vi "pick 1 ball new.vi"   [LabVIEW 2016, in "Test2.lvrbt"]
uses:
  Test2.lvrbt
  <vilib>/NXT/Hardware/Plugins/Tetrix DC Motor/TetrixDCMotorAddress.ctl
  <vilib>/NXT/Hardware/Plugins/Tetrix 180 deg Servo/Tetrix180ServoAddress.ctl
  <vilib>/NXT/Block Support/NXT_InputPort.ctl
  <vilib>/NXT/NXTIO Xnodes/NXTIONodeSubVIs/TETRIX IO Move Servos.vi
  <vilib>/NXT/Dual Mode Library/Waits/Wait_Num.vi
  <vilib>/NXT/NXTIO Xnodes/NXTIONodeSubVIs/TETRIX IO Move DC Motors.vi
  <vilib>/NXT/Dual Mode Library/Waits/Wait_EV3_Ultrasonic_Centimeters_Further.vi
  <vilib>/NXT/NXTIO Xnodes/NXTIONodeSubVIs/TETRIX IO Stop DC Motors.vi
  <vilib>/NXT/Dual Mode Library/Waits/Wait_EV3_Ultrasonic_Centimeter_Closer.vi
  <vilib>/NXT/NXTIO Xnodes/AddressXNode/NXTIOAddress.xnode
  <vilib>/NXT/Subs/LVHSConnector.ctl
  <vilib>/NXT/NXTIO Xnodes/NXTIOXNode/NXTIO.xnode
  <vilib>/NXT/LegoClasses/BrickReference/BrickReference.lvclass
types:
  T1 = typedef "Tetrix180ServoAddress.ctl" = i32
  T2 = cluster{"Tetrix180Servo":T1, "Tetrix180Servo":T1, "Tetrix180Servo":T1, "Tetrix180Servo":T1, "Tetrix180Servo":T1, "Tetrix180Servo":T1}
  T3 = typedef "LVHSConnector.ctl" = refnum<class "BrickReference.lvclass">
  T4 = typedef "TetrixDCMotorAddress.ctl" = i32
  T5 = typedef "NXT_InputPort.ctl" = u32
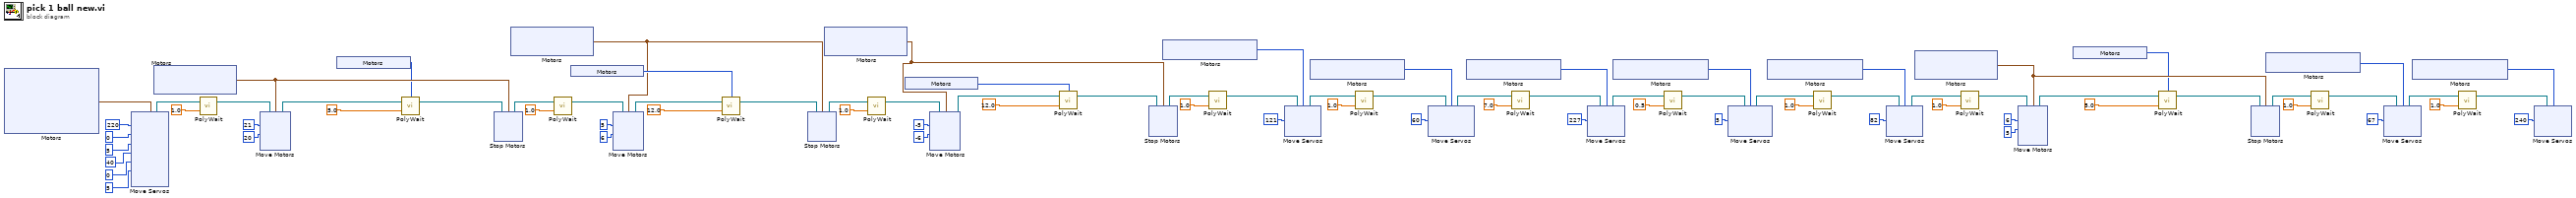
[diagram p0: block diagram]
diagram:
  n1 = xnode "Motors"() -> ("Motor"=w63:T2)
  n2 = xnode "Move Servos"("Position 6"=u8 5, "Position 5"=u8 0, "Position 4"=u8 40, "Position 3"=u8 5, "Position 2"=u8 0, "Position 1"=u8 220, "Motors"=w63) -> ("NXT/EV3"=w31:T3)  [unwired: 1 in]
  n3 = xnode "Motors"() -> ("Motor"=w33:cluster{"TetrixDCMotor":T4, "TetrixDCMotor":T4})
  n4 = call-poly <vilib>:"PolyWait.vi"("Time (1 sec)"=sgl 1.0, "NXT/EV3"=w31) -> ("NXT/EV3"=w30:T3)  [unwired: 2 in]
  n5 = xnode "Move Motors"("Power/Speed 2"=i8 20, "Power/Speed 1"=i8 21, "Motors"=w33, "NXT/EV3"=w30) -> ("NXT/EV3"=w36:T3)
  n6 = xnode "Motors"() -> ("Sensor"=w2:T5)
  n7 = call-poly <vilib>:"PolyWait.vi"("Centimeters (50)"=sgl 5.0, "NXT/EV3"=w36, "Port (Port 1)"=w2) -> ("NXT/EV3"=w34:T3)  [unwired: 1 in]
  n8 = xnode "Stop Motors"("Motors"=w33, "NXT/EV3"=w34) -> ("NXT/EV3"=w4:T3)
  n9 = xnode "Motors"() -> ("Motor"=w18:cluster{"TetrixDCMotor":T4, "TetrixDCMotor":T4})
  n10 = call-poly <vilib>:"PolyWait.vi"("Time (1 sec)"=sgl 1.0, "NXT/EV3"=w4) -> ("NXT/EV3"=w17:T3)  [unwired: 2 in]
  n11 = xnode "Motors"() -> ("Sensor"=w20:T5)
  n12 = xnode "Move Motors"("Power/Speed 2"=i8 6, "Power/Speed 1"=i8 5, "Motors"=w18, "NXT/EV3"=w17) -> ("NXT/EV3"=w22:T3)
  n13 = call-poly <vilib>:"PolyWait.vi"("Centimeters (40)"=sgl 12.0, "NXT/EV3"=w22, "Port (Port 1)"=w20) -> ("NXT/EV3"=w19:T3)  [unwired: 1 in]
  n14 = xnode "Stop Motors"("Motors"=w18, "NXT/EV3"=w19) -> ("NXT/EV3"=w16:T3)
  n15 = xnode "Motors"() -> ("Motor"=w9:cluster{"TetrixDCMotor":T4, "TetrixDCMotor":T4})
  n16 = call-poly <vilib>:"PolyWait.vi"("Time (1 sec)"=sgl 1.0, "NXT/EV3"=w16) -> ("NXT/EV3"=w12:T3)  [unwired: 2 in]
  n17 = xnode "Motors"() -> ("Sensor"=w7:T5)
  n18 = xnode "Move Motors"("Power/Speed 2"=i8 -6, "Power/Speed 1"=i8 -5, "Motors"=w9, "NXT/EV3"=w12) -> ("NXT/EV3"=w11:T3)
  n19 = call-poly <vilib>:"PolyWait.vi"("Centimeters (50)"=sgl 12.0, "NXT/EV3"=w11, "Port (Port 1)"=w7) -> ("NXT/EV3"=w10:T3)  [unwired: 1 in]
  n20 = xnode "Stop Motors"("Motors"=w9, "NXT/EV3"=w10) -> ("NXT/EV3"=w5:T3)
  n21 = xnode "Motors"() -> ("Motor"=w29:T1)
  n22 = call-poly <vilib>:"PolyWait.vi"("Time (1 sec)"=sgl 1.0, "NXT/EV3"=w5) -> ("NXT/EV3"=w3:T3)  [unwired: 2 in]
  n23 = xnode "Move Servos"("Position 1"=u8 121, "Motors"=w29, "NXT/EV3"=w3) -> ("NXT/EV3"=w27:T3)
  n24 = xnode "Motors"() -> ("Motor"=w75:T1)
  n25 = call-poly <vilib>:"PolyWait.vi"("Time (1 sec)"=sgl 1.0, "NXT/EV3"=w27) -> ("NXT/EV3"=w50:T3)  [unwired: 2 in]
  n26 = xnode "Move Servos"("Position 1"=u8 60, "Motors"=w75, "NXT/EV3"=w50) -> ("NXT/EV3"=w72:T3)
  n27 = xnode "Motors"() -> ("Motor"=w71:T1)
  n28 = call-poly <vilib>:"PolyWait.vi"("Time (1 sec)"=sgl 7.0, "NXT/EV3"=w72) -> ("NXT/EV3"=w69:T3)  [unwired: 2 in]
  n29 = xnode "Move Servos"("Position 1"=u8 227, "Motors"=w71, "NXT/EV3"=w69) -> ("NXT/EV3"=w67:T3)
  n30 = xnode "Motors"() -> ("Motor"=w66:T1)
  n31 = call-poly <vilib>:"PolyWait.vi"("Time (1 sec)"=sgl 0.5, "NXT/EV3"=w67) -> ("NXT/EV3"=w64:T3)  [unwired: 2 in]
  n32 = xnode "Move Servos"("Position 1"=u8 5, "Motors"=w66, "NXT/EV3"=w64) -> ("NXT/EV3"=w56:T3)
  n33 = xnode "Motors"() -> ("Motor"=w54:T1)
  n34 = call-poly <vilib>:"PolyWait.vi"("Time (1 sec)"=sgl 1.0, "NXT/EV3"=w56) -> ("NXT/EV3"=w53:T3)  [unwired: 2 in]
  n35 = xnode "Move Servos"("Position 1"=u8 82, "Motors"=w54, "NXT/EV3"=w53) -> ("NXT/EV3"=w52:T3)
  n36 = xnode "Motors"() -> ("Motor"=w78:cluster{"TetrixDCMotor":T4, "TetrixDCMotor":T4})
  n37 = call-poly <vilib>:"PolyWait.vi"("Time (1 sec)"=sgl 1.0, "NXT/EV3"=w52) -> ("NXT/EV3"=w76:T3)  [unwired: 2 in]
  n38 = xnode "Move Motors"("Power/Speed 2"=i8 5, "Power/Speed 1"=i8 6, "Motors"=w78, "NXT/EV3"=w76) -> ("NXT/EV3"=w80:T3)
  n39 = xnode "Motors"() -> ("Sensor"=w1:T5)
  n40 = call-poly <vilib>:"PolyWait.vi"("Centimeters (50)"=sgl 5.0, "NXT/EV3"=w80, "Port (Port 1)"=w1) -> ("NXT/EV3"=w79:T3)  [unwired: 1 in]
  n41 = xnode "Stop Motors"("Motors"=w78, "NXT/EV3"=w79) -> ("NXT/EV3"=w47:T3)
  n42 = xnode "Motors"() -> ("Motor"=w45:T1)
  n43 = call-poly <vilib>:"PolyWait.vi"("Time (1 sec)"=sgl 1.0, "NXT/EV3"=w47) -> ("NXT/EV3"=w44:T3)  [unwired: 2 in]
  n44 = xnode "Move Servos"("Position 1"=u8 67, "Motors"=w45, "NXT/EV3"=w44) -> ("NXT/EV3"=w42:T3)
  n45 = xnode "Motors"() -> ("Motor"=w40:T1)
  n46 = call-poly <vilib>:"PolyWait.vi"("Time (1 sec)"=sgl 1.0, "NXT/EV3"=w42) -> ("NXT/EV3"=w39:T3)  [unwired: 2 in]
  n47 = xnode "Move Servos"("Position 1"=u8 240, "Motors"=w40, "NXT/EV3"=w39) -> ()  [unwired: 1 out]
